vi "load tdms image from file.vi"() -> ()   [LabVIEW 2020]
panel:
  out "channel name out":string
  out "data 3":i32
  out "property names":string[](array[string])
  out "property values":variant[](array[variant])
  out "channel names":string[](array[string])
  out "found 2":bool
  out "found":bool
  out "data 2":i32
  out "size(s)":i32
  out "Intensity Graph":u16[][](graph)
  out "time to read":u32
  in  "file path":path
  out "data":u16[](array[numeric])
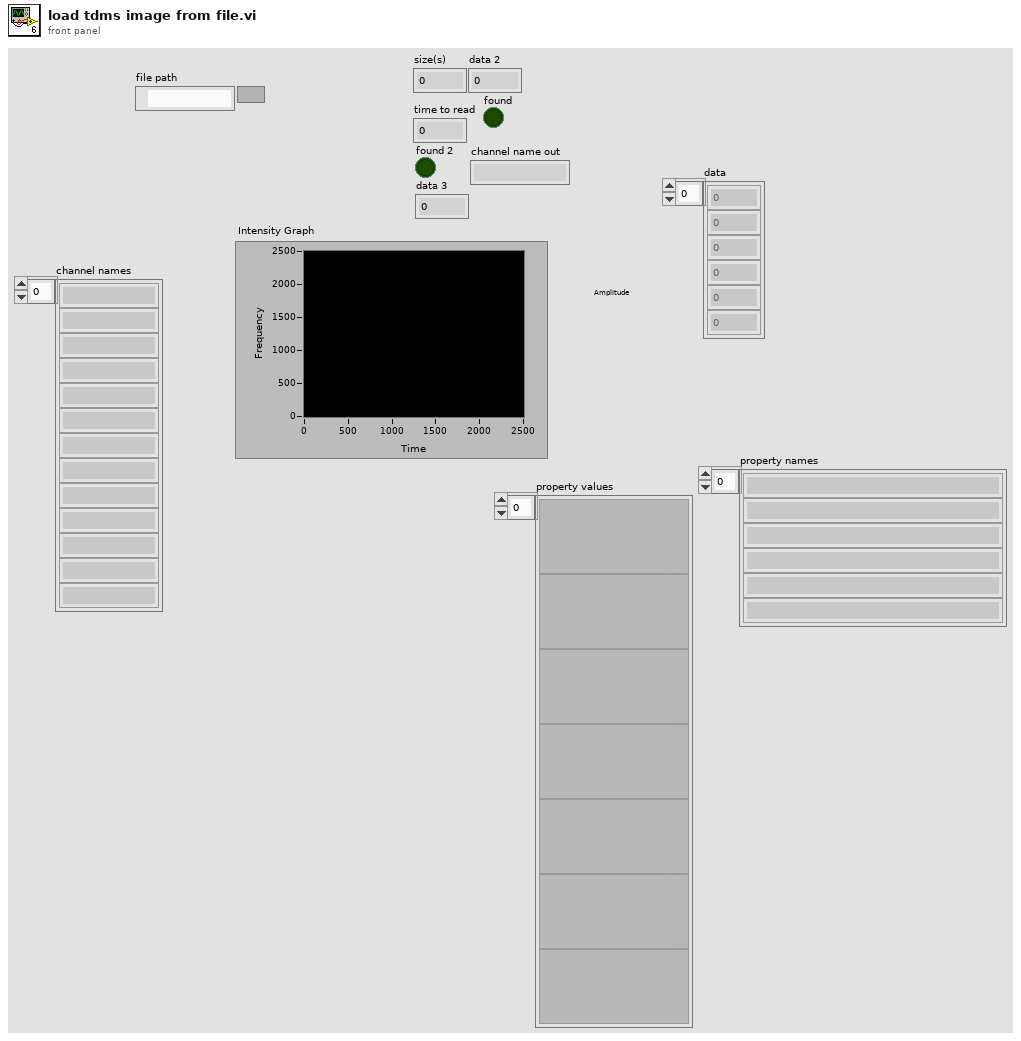
[diagram p1: front panel]
types:
  T1 = enum16{"open", "open or create", "create or replace", "create", "open (read-only)"}
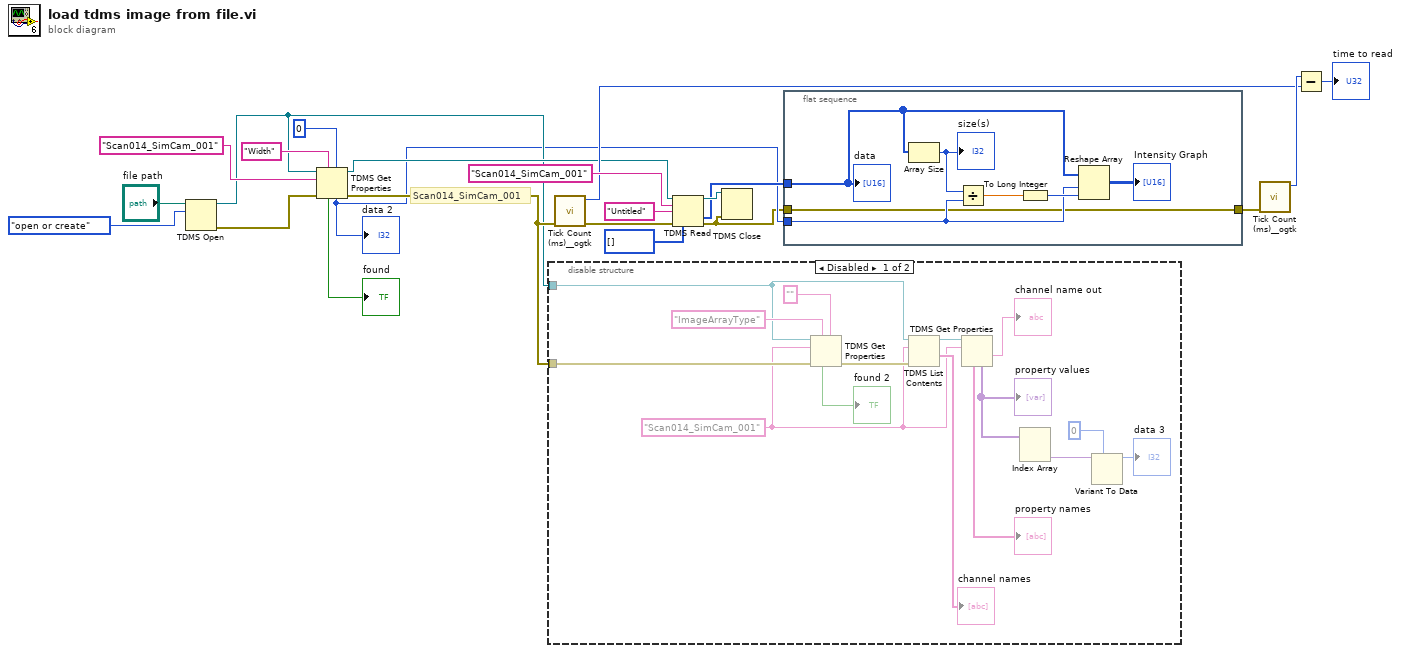
[diagram p0: block diagram]
diagram:
  # "Scan014_SimCam_001"
  n1 = TDMS Open(10:T1."open or create" ("operation (0:open)"), 11:"file path") -> (0:w12:errorcluster, 3:w4:refnum<k34>)  [unwired: 5 in]
  n2 = TDMS Get Properties(5:0 ("x"), 7:"Width", 8:w12, 10:"Scan014_SimCam_001" ("group name in"), 11:w4) -> (0:w5:errorcluster, 3:w6:refnum<k34>, 4:w3:i32, 6:→"found":bool)  [unwired: 1 in, 2 out]
  "data 2" <- w3
  n3 = disable-structure shown="Disabled" {
    disable-tunnel: w5 -> [w36 _]
    disable-tunnel: w4 -> [w33 _]
    frame Disabled {
      w29 = "Scan014_SimCam_001" ("group name in")
      n4 = TDMS Get Properties(5:"" ("data type"), 7:"ImageArrayType", 8:w36, 10:w29, 11:w33) -> (0:w32:errorcluster, 6:→"found 2":bool)  [unwired: 1 in, 4 out]
      n5 = TDMS List Contents(4:w32, 6:w29, 7:w33) -> (1:→"channel names":string[], 3:w30:refnum<k34>)  [unwired: 2 out]
      n6 = TDMS Get Properties(10:w29, 11:w30) -> (1:→"channel name out":string, 4:w27:variant[], 6:→"property names":string[])  [unwired: 4 in, 3 out]
      "property values" <- w27
      n7 = Index Array(array=w27) -> (element #2=w23:variant)  [unwired: 2 in, 1 out]
      n8 = Variant To Data(type=0, Variant=w23) -> (data=→"data 3":i32)  [unwired: 1 in, 1 out]
    }
    frame Enabled {
    }
  }
  n9 = call <userlib>:"Tick Count (ms)__ogtk.vi"("error in (no error)"=w5) -> ("error out"=w18:errorcluster, "millisecond timer value"=w16:u32)  [unwired: 9 in]
  n10 = TDMS Read(0:w6, 5:"Scan014_SimCam_001" ("group name in"), 7:"Untitled" ("channel name(s) in"), 11:w18, 12:u16[] [] ("output array")) -> (4:w15:refnum<k34>, 10:w8:u16[], 15:w2:errorcluster)  [unwired: 3 in, 3 out]
  n11 = TDMS Close(8:w2, 11:w15) -> ()  [unwired: 2 out]
  n12 = flat-sequence {
    tunnel: w8 -> [w44]
    tunnel: w3 -> [w39]
    tunnel: w2 -> [w38]
    tunnel: [w38] -> w1
    frame #0 {
      n13 = Array Size(array=w44) -> (size(s)=w43:i32)
      "size(s)" <- w43
      n14 = Divide(x=w43, y=w39) -> (x/y=w42:dbl)
      n15 = To Long Integer(number=w42) -> (32bit integer=w41:i32)
      n16 = Reshape Array(w44, w39, w41) -> (→"Intensity Graph":u16[][])
      "data" <- w44
    }
  }
  n17 = call <userlib>:"Tick Count (ms)__ogtk.vi"("error in (no error)"=w1) -> ("millisecond timer value"=w17:u32)  [unwired: 9 in, 1 out]
  n18 = Subtract(x=w17, y=w16) -> (x-y=→"time to read":u32)
